vi "GetColorPlanes.vi"(11 "image data":T1) -> (0 "Grey":T1, 1 "Blue":T1, 2 "Green":T1, 3 "Red":T1)   [LabVIEW 2019]
uses:
  <vilib>/picture/picture.llb/imagedata.ctl
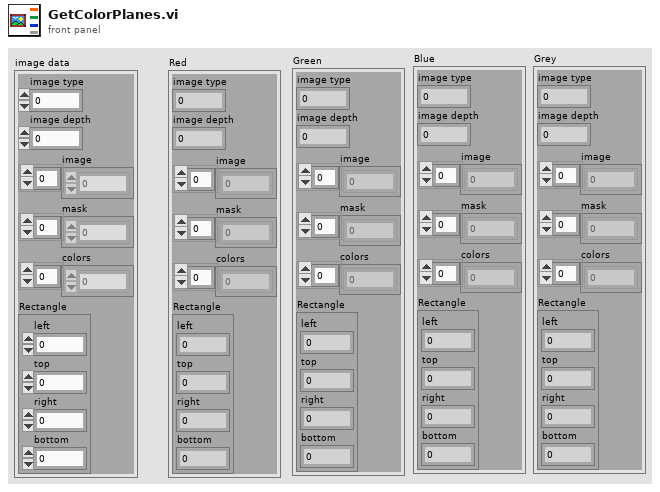
[diagram p1: front panel]
types:
  T1 = typedef "imagedata.ctl" = cluster{"image type":i32, "image depth":i32, "image":u8[], "mask":u8[], "colors":u32[], "Rectangle":cluster{"left":i16, "top":i16, "right":i16, "bottom":i16}}
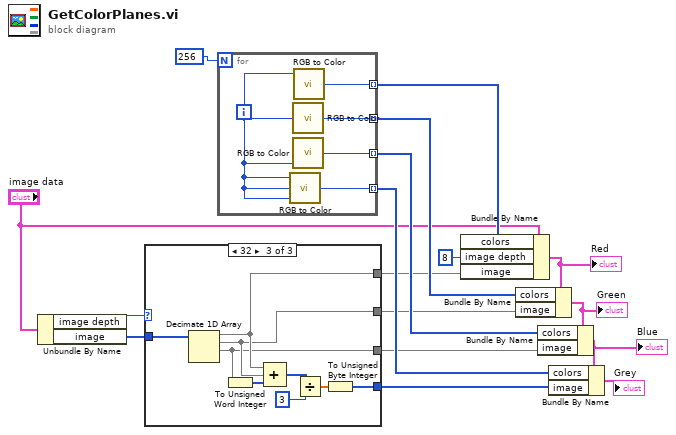
[diagram p0: block diagram]
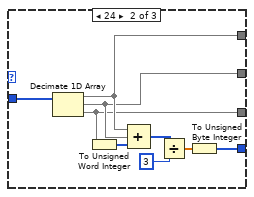
[diagram p3: hidden frame]
diagram:
  n1 = Unbundle By Name("image data") -> ("image depth"=w1:i32, "image"=w2:u8[])
  n2 = case shown="32" w1 {
    tunnel: w2 -> [w18 w27 w36]
    tunnel: [w18 w26 w35] -> w4
    tunnel: [w18 w25 w34] -> w6
    tunnel: [w18 w24 w33] -> w7
    tunnel: [w18 w20 w29] -> w8
    frame 0, Default {
    }
    frame 24 {
      n3 = Decimate 1D Array(w27) -> (w26:u8[], w25:u8[], w24:u8[])
      n4 = To Unsigned Word Integer(number=w24) -> (unsigned 16bit integer=w19:u16[])
      n5 = Compound Arithmetic op=ADD(w26, w25, w19) -> (w23:u16[])
      n6 = Divide(x=w23, y=3) -> (x/y=w21:dbl[])
      n7 = To Unsigned Byte Integer(number=w21) -> (unsigned 8bit integer=w20:u8[])
    }
    frame 32 {
      n8 = Decimate 1D Array(w36) -> (w35:u8[], w34:u8[], w33:u8[])  [unwired: 1 out]
      n9 = To Unsigned Word Integer(number=w33) -> (unsigned 16bit integer=w28:u16[])
      n10 = Compound Arithmetic op=ADD(w35, w34, w28) -> (w32:u16[])
      n11 = Divide(x=w32, y=3) -> (x/y=w30:dbl[])
      n12 = To Unsigned Byte Integer(number=w30) -> (unsigned 8bit integer=w29:u8[])
    }
  }
  n13 = for {
    N: 256 -> [_]
    tunnel: [w40] -> w11 mode=indexing
    tunnel: [w39] -> w12 mode=indexing
    tunnel: [w38] -> w13 mode=indexing
    tunnel: [w37] -> w14 mode=indexing
    i -> [w41]
    n14 = call <vilib>:"RGB to Color.vi"("B"=w41, "G"=w41, "R"=w41) -> ("Color"=w39:u32)
    n15 = call <vilib>:"RGB to Color.vi"("G"=w41) -> ("Color"=w37:u32)  [unwired: 2 in]
    n16 = call <vilib>:"RGB to Color.vi"("B"=w41) -> ("Color"=w38:u32)  [unwired: 2 in]
    n17 = call <vilib>:"RGB to Color.vi"("R"=w41) -> ("Color"=w40:u32)  [unwired: 2 in]
  }
  n18 = Bundle By Name(cluster="image data", "colors"=w11, "image depth"=8, "image"=w4) -> (w17:T1)
  "Red" <- w17
  n19 = Bundle By Name(cluster=w17, "colors"=w14, "image"=w6) -> (w15:T1)
  "Green" <- w15
  n20 = Bundle By Name(cluster=w15, "colors"=w13, "image"=w7) -> (w16:T1)
  "Blue" <- w16
  n21 = Bundle By Name(cluster=w16, "colors"=w12, "image"=w8) -> (→"Grey":T1)
